vi "new_XY_deviation_angle(double).vi"(0 "KNR in":T2, 1 "配對數":i32, 5 "Circles (Shape Detection 1)":T1(array[cluster]) {"Position"."Y" format="%.2f"; "Position"."X" format="%.2f"}, 7 "ふ计":i32, 11 "Error":errorcluster) -> (4 "KNR out":T2, 6 "X":dbl, 8 "Y":dbl, 10 "角度":dbl, 15 "error out":errorcluster)   [LabVIEW 2013]
uses:
  <userlib>/KNR OS 3.0 LabVIEW Toolkit/Type Definition/KNR3 Reference.ctl
  <userlib>/_FPGA Interface Advanced Tools/FPGA Interface Base/FPGA Interface Base.lvclass
  <userlib>/KNR OS 3.0 LabVIEW Toolkit/Type Definition/Resource.ctl
panel:
  out "Y中心":sgl
  out "Center_XY陣列(由小到大)":cluster{"X":sgl, "Y":sgl}[](array[cluster])
  out "L0 - L1":sgl
  out "L0 - L2":sgl
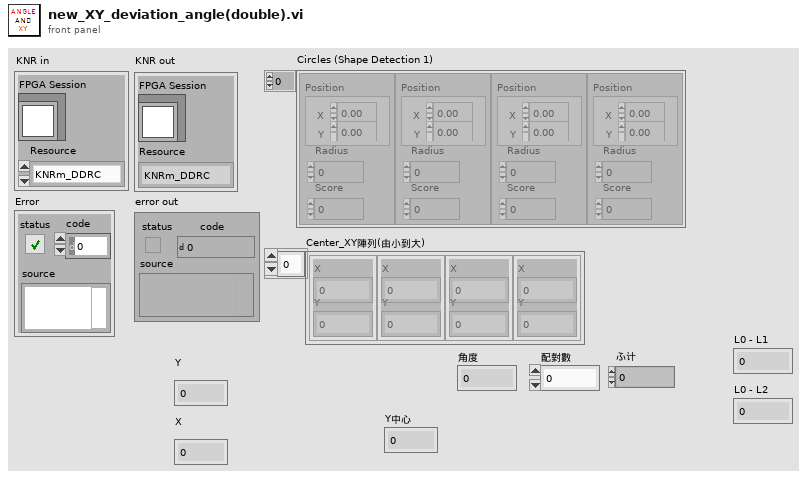
[diagram p1: front panel]
types:
  T1 = cluster{"Position":cluster{"X":sgl, "Y":sgl}, "Radius":dbl, "Score":dbl}[]
  T2 = typedef "KNR3 Reference.ctl" = cluster{"FPGA Session":refnum<class "FPGA Interface Base.lvclass">, "Resource":T3}
  T3 = typedef "Resource.ctl" = enum16{"KNRm_DDRC", "KNRm_DDDD", "KNRm_DDDR", "KNRm_DDDC", "KNR"}
  T4 = cluster{"Position":cluster{"X":sgl, "Y":sgl}, "Radius":dbl, "Score":dbl}
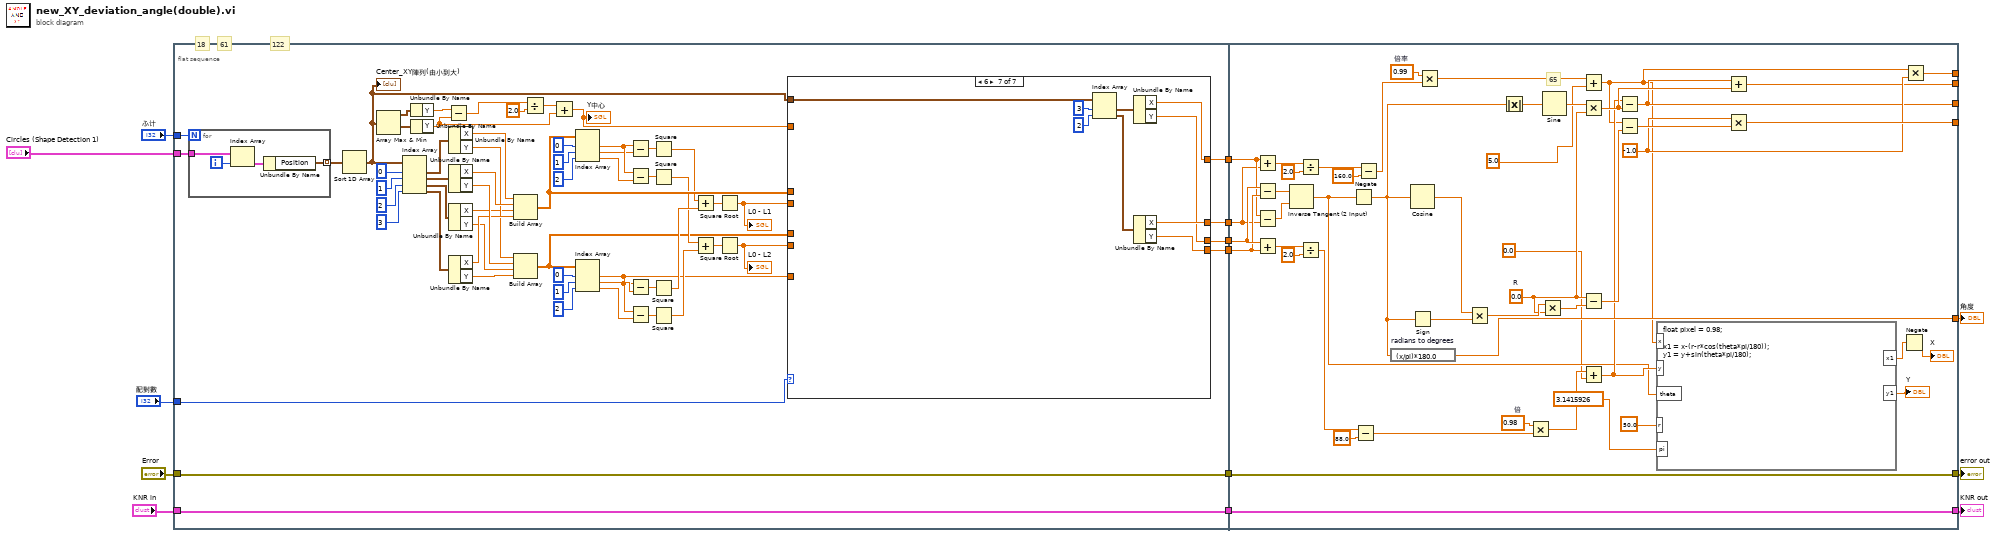
[diagram p0: block diagram]
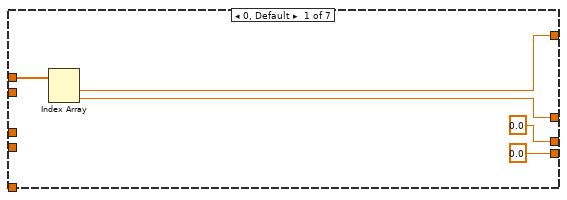
[diagram p2: hidden frame]
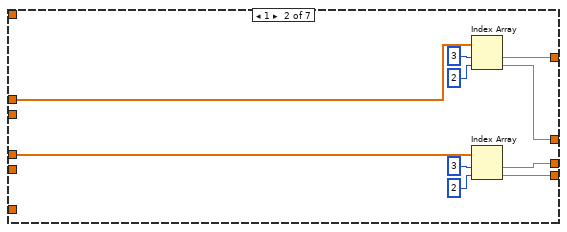
[diagram p3: hidden frame]
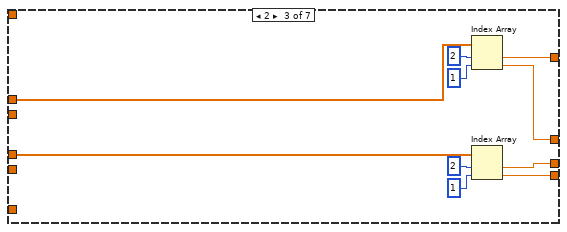
[diagram p4: hidden frame]
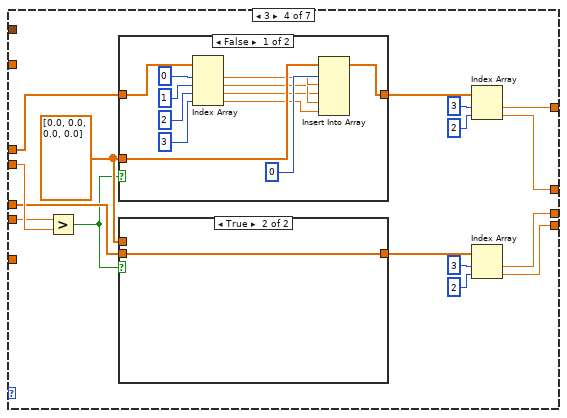
[diagram p5: hidden frame]
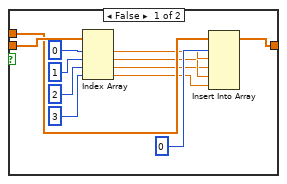
[diagram p6: hidden frame]
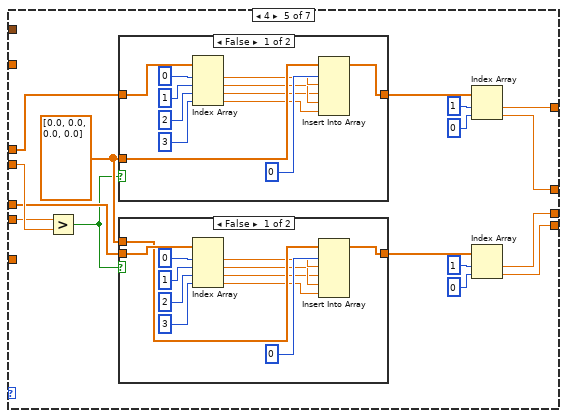
[diagram p8: hidden frame]
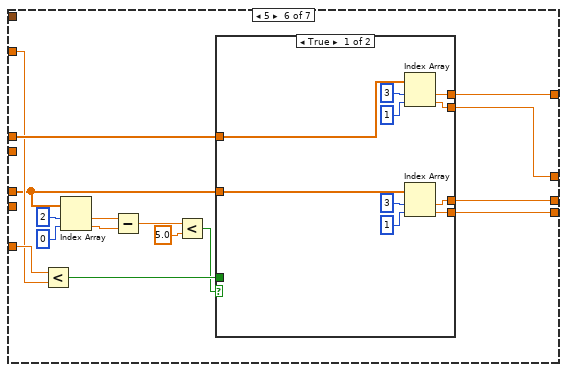
[diagram p11: hidden frame]
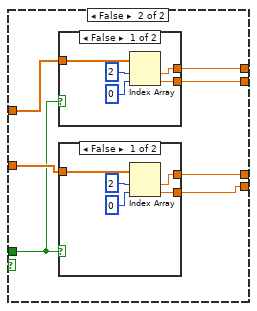
[diagram p12: hidden frame]
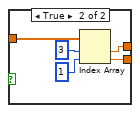
[diagram p13: hidden frame]
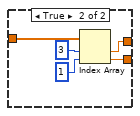
[diagram p14: hidden frame]
diagram:
  # "122"
  # "61"
  # "18"
  n1 = flat-sequence {
    tunnel: "KNR in" -> [w69]
    tunnel: "Error" -> [w70]
    tunnel: "ふ计" -> [w68]
    tunnel: "Circles (Shape Detection 1)" -> [w67]
    tunnel: [w70] -> w14
    tunnel: [w69] -> w13
    tunnel: "配對數" -> [w22]
    tunnel: [w26] -> w12
    tunnel: [w25] -> w11
    tunnel: [w24] -> w10
    tunnel: [w23] -> w9
    tunnel: [w298] -> w5
    tunnel: [w299] -> w6
    tunnel: w14 -> [w299]
    tunnel: w13 -> [w298]
    tunnel: w12 -> [w286]
    tunnel: w11 -> [w285]
    tunnel: w10 -> [w295]
    tunnel: w9 -> [w294]
    tunnel: [w289] -> w1
    tunnel: [w262] -> _
    tunnel: [w271] -> _
    tunnel: [w265] -> _
    tunnel: [w263] -> _
    frame #0 {
      n2 = for {
        N: w68 -> [_]
        tunnel: w67 -> [w250]
        tunnel: [w249] -> w75 mode=indexing
        i -> [w248]
        n3 = Index Array(array=w250, index=w248) -> (element=w247:T4)
        n4 = Unbundle By Name(w247) -> ("Position"=w249:cluster{"X":sgl, "Y":sgl})
      }
      n5 = Sort 1D Array(array=w75) -> (sorted array=w30:cluster{"X":sgl, "Y":sgl}[])
      "Center_XY陣列(由小到大)" <- w30
      n6 = Array Max & Min(array=w30) -> (max value=w31:cluster{"X":sgl, "Y":sgl}, min value=w32:cluster{"X":sgl, "Y":sgl})  [unwired: 2 out]
      n7 = Index Array(array=w30, index #1=0 ("index"), index #2=1 ("index"), index #3=2 ("index"), index #4=3 ("index")) -> (element #1=w65:cluster{"X":sgl, "Y":sgl}, element #2=w64:cluster{"X":sgl, "Y":sgl}, element #3=w63:cluster{"X":sgl, "Y":sgl}, element #4=w62:cluster{"X":sgl, "Y":sgl})
      n8 = Unbundle By Name(w31) -> ("Y"=w33:sgl)
      n9 = Unbundle By Name(w32) -> ("Y"=w36:sgl)
      n10 = Subtract(x=w33, y=w36) -> (x-y=w37:sgl)
      n11 = Unbundle By Name(w65) -> ("X"=w21:sgl, "Y"=w18:sgl)
      n12 = Unbundle By Name(w64) -> ("X"=w20:sgl, "Y"=w66:sgl)
      n13 = Unbundle By Name(w63) -> ("X"=w17:sgl, "Y"=w16:sgl)
      n14 = Unbundle By Name(w62) -> ("X"=w19:sgl, "Y"=w15:sgl)
      n15 = Build Array(w21, w20, w17, w19) -> (w54:sgl[])
      n16 = Build Array(w18, w66, w16, w15) -> (w28:sgl[])
      n17 = Divide(x=w37, y=sgl 2.0) -> (x/y=w35:sgl)
      n18 = Add(x=w35, y=w36) -> (x+y=w29:sgl)
      "Y中心" <- w29
      n19 = Index Array(array=w54, index #1=0 ("index"), index #2=1 ("index"), index #3=2 ("index")) -> (element #1=w40:sgl, element #2=w38:sgl, element #3=w39:sgl)
      n20 = Index Array(array=w28, index #1=0 ("index"), index #2=1 ("index"), index #3=2 ("index")) -> (element #1=w27:sgl, element #2=w42:sgl, element #3=w41:sgl)
      n21 = Subtract(x=w40, y=w38) -> (x-y=w53:sgl)
      n22 = Subtract(x=w40, y=w39) -> (x-y=w52:sgl)
      n23 = Subtract(x=w27, y=w42) -> (x-y=w44:sgl)
      n24 = Subtract(x=w27, y=w41) -> (x-y=w58:sgl)
      n25 = Square(x=w53) -> (x^2=w51:sgl)
      n26 = Square(x=w52) -> (x^2=w48:sgl)
      n27 = Square(x=w44) -> (x^2=w50:sgl)
      n28 = Square(x=w58) -> (x^2=w43:sgl)
      n29 = Add(x=w51, y=w50) -> (x+y=w45:sgl)
      n30 = Add(x=w48, y=w43) -> (x+y=w47:sgl)
      n31 = Square Root(x=w45) -> (sqrt(x)=w49:sgl)
      "L0 - L1" <- w49
      n32 = Square Root(x=w47) -> (sqrt(x)=w46:sgl)
      "L0 - L2" <- w46
      n33 = case shown="6" w22 {
        tunnel: w54 -> [w80 w90 w100 w114 w156 w198 _]
        tunnel: [w79 w87 w98 w115 w157 w200 w243] -> w26
        tunnel: w30 -> [_ _ _ _ _ _ w245]
        tunnel: w28 -> [_ w85 w93 w103 w145 w191 _]
        tunnel: [w78 w86 w96 w112 w152 w199 w240] -> w25
        tunnel: w49 -> [_ _ _ w111 w155 _ _]
        tunnel: w46 -> [_ _ _ w110 w154 _ _]
        tunnel: w27 -> [_ _ _ _ _ w197 _]
        tunnel: w29 -> [_ _ _ _ _ w196 _]
        tunnel: [0.0 w82 w92 w106 w148 w194 w238] -> w24
        tunnel: [0.0 w81 w91 w105 w147 w193 w239] -> w23
        frame 0, Default {
          n34 = Index Array(array=w80) -> (element #1=w79:sgl, element #2=w78:sgl)  [unwired: 2 in]
        }
        frame 1 {
          n35 = Index Array(array=w90, index #1=3 ("index"), index #2=2 ("index")) -> (element #1=w87:sgl, element #2=w86:sgl)
          n36 = Index Array(array=w85, index #1=3 ("index"), index #2=2 ("index")) -> (element #1=w82:sgl, element #2=w81:sgl)
        }
        frame 2 {
          n37 = Index Array(array=w100, index #1=2 ("index"), index #2=1 ("index")) -> (element #1=w98:sgl, element #2=w96:sgl)
          n38 = Index Array(array=w93, index #1=2 ("index"), index #2=1 ("index")) -> (element #1=w92:sgl, element #2=w91:sgl)
        }
        frame 3 {
          w102 = dbl[] [0.0, 0.0, 0.0, 0.0]
          n39 = Greater?(x=w110, y=w111) -> (0:w101:bool)
          n40 = case shown="False" w101 {
            tunnel: w114 -> [w137 w142]
            tunnel: w102 -> [w136 _]
            tunnel: [w130 w142] -> w109
            frame False {
              n41 = Index Array(array=w137, index #1=0 ("index"), index #2=1 ("index"), index #3=2 ("index"), index #4=3 ("index")) -> (element #1=w134:sgl, element #2=w132:sgl, element #3=w131:sgl, element #4=w133:sgl)
              n42 = Insert Into Array(array=w136, index=0, new element #1=w134, new element #2=w131, new element #3=w132, new element #4=w133) -> (w130:dbl[])
            }
            frame True {
            }
          }
          n43 = case shown="True" w101 {
            tunnel: w103 -> [w124 w129]
            tunnel: w102 -> [w123 _]
            tunnel: [w117 w129] -> w104
            frame False {
              n44 = Index Array(array=w124, index #1=0 ("index"), index #2=1 ("index"), index #3=2 ("index"), index #4=3 ("index")) -> (element #1=w121:sgl, element #2=w119:sgl, element #3=w118:sgl, element #4=w120:sgl)
              n45 = Insert Into Array(array=w123, index=0, new element #1=w121, new element #2=w118, new element #3=w119, new element #4=w120) -> (w117:dbl[])
            }
            frame True {
            }
          }
          n46 = Index Array(array=w109, index #1=3 ("index"), index #2=2 ("index")) -> (element #1=w115:dbl, element #2=w112:dbl)
          n47 = Index Array(array=w104, index #1=3 ("index"), index #2=2 ("index")) -> (element #1=w106:dbl, element #2=w105:dbl)
        }
        frame 4 {
          w144 = dbl[] [0.0, 0.0, 0.0, 0.0]
          n48 = Greater?(x=w154, y=w155) -> (0:w143:bool)
          n49 = case shown="False" w143 {
            tunnel: w156 -> [w179 w184]
            tunnel: w144 -> [w178 _]
            tunnel: [w172 w184] -> w149
            frame False {
              n50 = Index Array(array=w179, index #1=0 ("index"), index #2=1 ("index"), index #3=2 ("index"), index #4=3 ("index")) -> (element #1=w176:sgl, element #2=w174:sgl, element #3=w173:sgl, element #4=w175:sgl)
              n51 = Insert Into Array(array=w178, index=0, new element #1=w176, new element #2=w173, new element #3=w174, new element #4=w175) -> (w172:dbl[])
            }
            frame True {
            }
          }
          n52 = case shown="False" w143 {
            tunnel: w145 -> [w166 w171]
            tunnel: w144 -> [w165 _]
            tunnel: [w159 w171] -> w146
            frame False {
              n53 = Index Array(array=w166, index #1=0 ("index"), index #2=1 ("index"), index #3=2 ("index"), index #4=3 ("index")) -> (element #1=w163:sgl, element #2=w161:sgl, element #3=w160:sgl, element #4=w162:sgl)
              n54 = Insert Into Array(array=w165, index=0, new element #1=w163, new element #2=w160, new element #3=w161, new element #4=w162) -> (w159:dbl[])
            }
            frame True {
            }
          }
          n55 = Index Array(array=w149, index #1=1 ("index"), index #2=0 ("index")) -> (element #1=w157:dbl, element #2=w152:dbl)
          n56 = Index Array(array=w146, index #1=1 ("index"), index #2=0 ("index")) -> (element #1=w148:dbl, element #2=w147:dbl)
        }
        frame 5 {
          n57 = Less?(x=w197, y=w196) -> (x < y?=w195:bool)
          n58 = Index Array(array=w191, index #1=2 ("index"), index #2=0 ("index")) -> (element #1=w188:sgl, element #2=w187:sgl)
          n59 = Subtract(x=w188, y=w187) -> (x-y=w186:sgl)
          n60 = Less?(x=w186, y=sgl 5.0) -> (x < y?=w192:bool)
          n61 = case shown="True" w192 {
            tunnel: [w209 w217] -> w200
            tunnel: [w208 w216] -> w199
            tunnel: w198 -> [w210 w215]
            tunnel: w191 -> [w206 w214]
            tunnel: w195 -> [_ w213]
            tunnel: [w207 w212] -> w194
            tunnel: [w205 w211] -> w193
            frame True {
              n62 = Index Array(array=w210, index #1=3 ("index"), index #2=1 ("index")) -> (element #1=w209:sgl, element #2=w208:sgl)
              n63 = Index Array(array=w206, index #1=3 ("index"), index #2=1 ("index")) -> (element #1=w207:sgl, element #2=w205:sgl)
            }
            frame False {
              n64 = case shown="False" w213 {
                tunnel: [w219 w226] -> w217
                tunnel: [w218 w224] -> w216
                tunnel: w215 -> [w220 w223]
                frame False {
                  n65 = Index Array(array=w220, index #1=2 ("index"), index #2=0 ("index")) -> (element #1=w219:sgl, element #2=w218:sgl)
                }
                frame True {
                  n66 = Index Array(array=w223, index #1=3 ("index"), index #2=1 ("index")) -> (element #1=w226:sgl, element #2=w224:sgl)
                }
              }
              n67 = case shown="False" w213 {
                tunnel: w214 -> [w228 w236]
                tunnel: [w230 w235] -> w212
                tunnel: [w229 w233] -> w211
                frame False {
                  n68 = Index Array(array=w228, index #1=2 ("index"), index #2=0 ("index")) -> (element #1=w230:sgl, element #2=w229:sgl)
                }
                frame True {
                  n69 = Index Array(array=w236, index #1=3 ("index"), index #2=1 ("index")) -> (element #1=w235:sgl, element #2=w233:sgl)
                }
              }
            }
          }
        }
        frame 6 {
          n70 = Index Array(array=w245, index #1=3 ("index"), index #2=2 ("index")) -> (element #1=w244:cluster{"X":sgl, "Y":sgl}, element #2=w241:cluster{"X":sgl, "Y":sgl})
          n71 = Unbundle By Name(w244) -> ("X"=w243:sgl, "Y"=w238:sgl)
          n72 = Unbundle By Name(w241) -> ("X"=w240:sgl, "Y"=w239:sgl)
        }
      }
    }
    frame #1 {
      w266 = -1.0 ("x")
      w275 = 0.98  # 倍
      w277 = 0.99  # 倍率
      w268 = 0.0  # R
      # "65"
      n73 = Add(x=w286, y=w285) -> (x+y=w284:dbl)
      n74 = Subtract(x=w295, y=w294) -> (x-y=w296:dbl)
      n75 = Subtract(x=w286, y=w285) -> (x-y=w297:dbl)
      n76 = Add(x=w295, y=w294) -> (x+y=w293:dbl)
      n77 = Inverse Tangent (2 Input)(1:w297, 2:w296) -> (0:w258:dbl)
      n78 = Divide(x=w284, y=2.0) -> (x/y=w281:dbl)
      n79 = Divide(x=w293, y=2.0) -> (x/y=w291:dbl)
      n80 = Negate(x=w258) -> (-x=w255:dbl)
      n81 = Subtract(x=w291, y=88.0) -> (x-y=w274:dbl)
      n82 = Subtract(x=w281, y=160.0) -> (x-y=w278:dbl)
      n83 = expression code="(x/pi)*180.0" "radians to degrees"(w255) -> (w289:dbl)
      n84 = Cosine(x=w255) -> (cos(x)=w270:dbl)
      n85 = Sign(1:w255) -> (0:w267:dbl)
      n86 = Multiply(x=w277, y=w278) -> (x*y=w276:dbl)
      n87 = Multiply(x=w270, y=w267) -> (x*y=w269:dbl)
      n88 = Absolute Value(x=w255) -> (abs(x)=w288:dbl)
      n89 = Multiply(x=w275, y=w274) -> (x*y=w273:dbl)
      n90 = Multiply(x=w269, y=w268) -> (x*y=w280:dbl)
      n91 = Sine(x=w288) -> (sin(x)=w287:dbl)
      n92 = Add(x=w276, y=5.0) -> (x+y=w259:dbl)
      n93 = Multiply(x=w287, y=w268) -> (x*y=w264:dbl)
      n94 = Subtract(x=w268, y=w280) -> (x-y=w279:dbl)
      n95 = Add(x=w273, y=0.0) -> (x+y=w260:dbl)
      n96 = Subtract(x=w260, y=w264) -> (x-y=w262:dbl)
      n97 = Subtract(x=w259, y=w279) -> (x-y=w272:dbl)
      n98 = formula code="float pixel = 0.98;\n\nx1 = x-(r-r*cos(theta*pi/180));\ny1 = y+sin(theta*pi/180);"("x"=w259, "y"=w260, "theta"=w258, "r"=50.0, "pi"=3.1415926) -> ("x1"=w252:dbl, "y1"=→"Y":dbl)
      n99 = Add(x=w262, y=w264) -> (x+y=w263:dbl)
      n100 = Multiply(x=w266, y=w272) -> (x*y=w271:dbl)
      n101 = Negate(x=w252) -> (-x=→"X":dbl)
      n102 = Multiply(x=w259, y=w266) -> (x*y=w265:dbl)
    }
  }
  "error out" <- w6
  "KNR out" <- w5
  "角度" <- w1
